vi "RegisterSettings.vi"(8 "error in":errorcluster, 11 "MainFGV_data":T1) -> (0 "error out":errorcluster, 3 "MainFGV_data out":T1)   [LabVIEW 2017]
uses:
  MainFGV_data.ctl
  CurrentMeter/CM_data.ctl
  CurrentMeter/CM_SerialNumber.ctl
  StrainGauge/SG_data.ctl
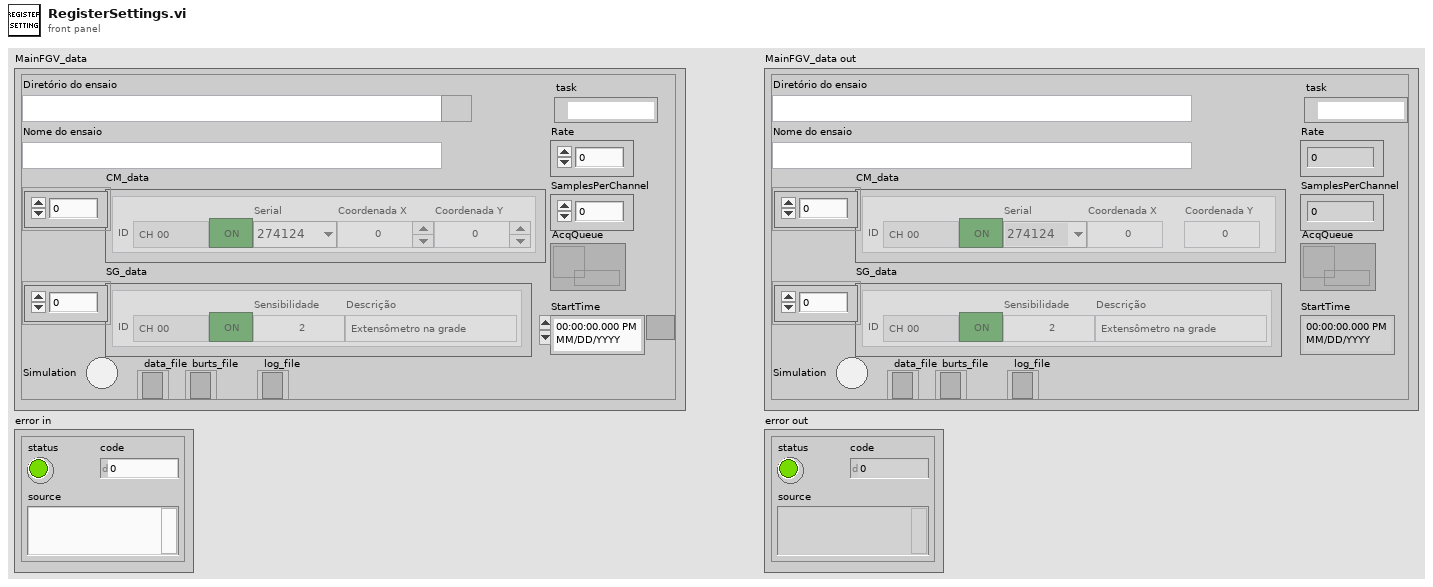
[diagram p1: front panel]
types:
  T1 = typedef "MainFGV_data.ctl" = cluster{"TestDir":path, "TestName":string, "CM_data":T2[], "SG_data":T4[], "Simulation":bool, "task":refnum<k21>, "data_file":refnum<file>, "burts_file":refnum<file>, "log_file":refnum<file>, "Rate":dbl, "SamplesPerChannel":dbl, "AcqQueue":refnum<queue>, "StartTime":timestamp}
  T2 = typedef "CM_data.ctl" = cluster{"Serial":T3, "Coordenada X":dbl, "Coordenada Y":dbl, "ID":string, "active":bool}
  T3 = typedef "CM_SerialNumber.ctl" = enum16{"274124", "274125", "274126", "274127", "274128"}
  T4 = typedef "SG_data.ctl" = cluster{"ID":string, "Sensibilidade":dbl, "Descrição":string, "active":bool}
  T5 = enum16{"open", "replace", "create", "open or create", "replace or create", "replace or create with confirmation"}
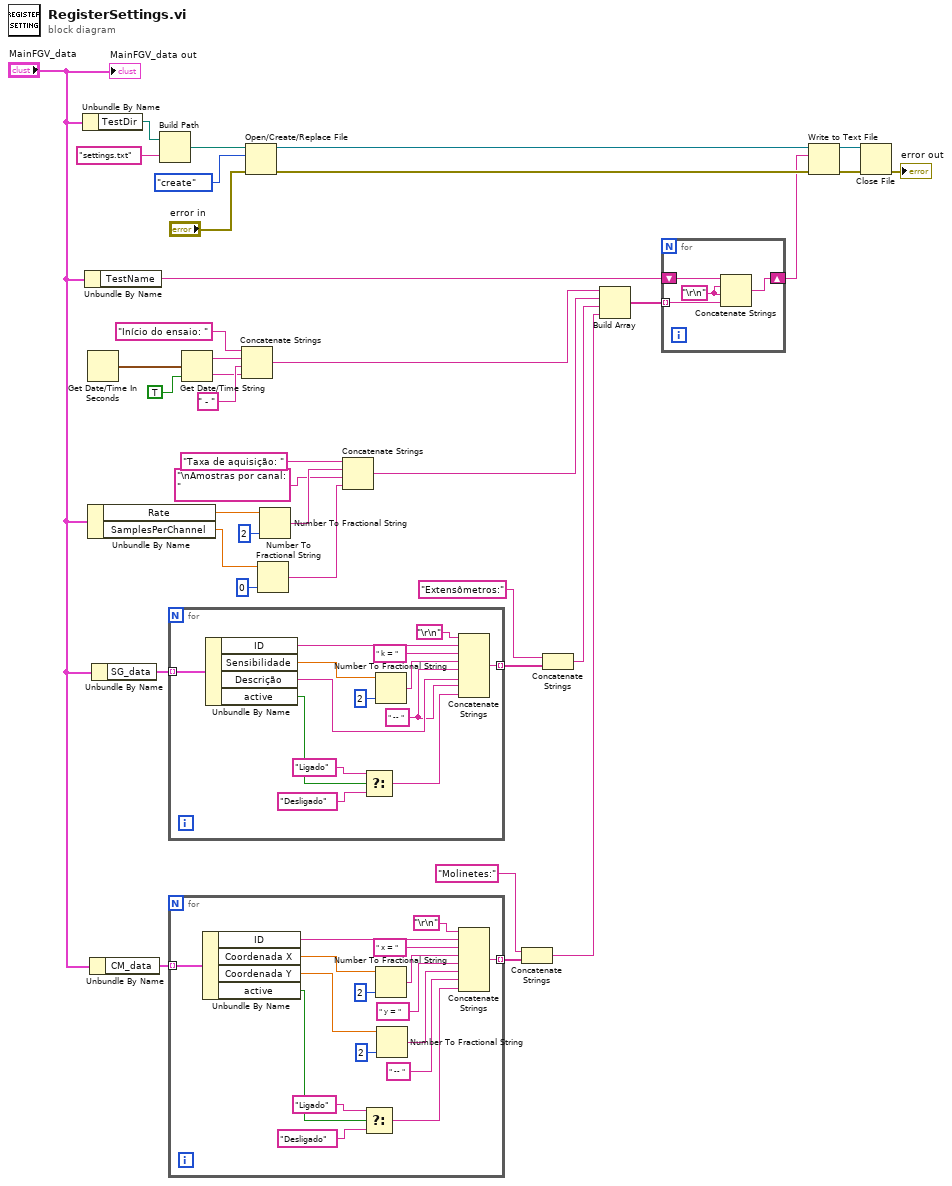
[diagram p0: block diagram]
diagram:
  n1 = Unbundle By Name("MainFGV_data") -> ("TestDir"=w38:path)
  n2 = Unbundle By Name("MainFGV_data") -> ("TestName"=w2:string)
  n3 = Get Date/Time In Seconds() -> (seconds since 1Jan1904=w1:timestamp)
  n4 = Unbundle By Name("MainFGV_data") -> ("Rate"=w28:dbl, "SamplesPerChannel"=w24:dbl)
  n5 = Unbundle By Name("MainFGV_data") -> ("CM_data"=w18:T2[])
  n6 = Unbundle By Name("MainFGV_data") -> ("SG_data"=w21:T4[])
  n7 = Build Path(base path=w38, name or relative path="settings.txt") -> (appended path=w36:path)
  n8 = for {
    tunnel: w21 -> [w52] mode=indexing
    tunnel: [w40] -> w20 mode=indexing
    w45 = " -- " ("string")
    n9 = Unbundle By Name(w52) -> ("ID"=w51:string, "Sensibilidade"=w48:dbl, "Descrição"=w46:string, "active"=w44:bool)
    n10 = Select(t="Ligado" ("string"), s=w44, f="Desligado" ("string")) -> (s? t:f=w41:string)
    n11 = Number To Fractional String(number=w48, precision (6)=i16 2) -> (F-format string=w47:string)  [unwired: 2 in]
    n12 = Concatenate Strings("\r\n", w51, " k = " ("string"), w47, w45, w46, w45, w41) -> (w40:string)
  }
  n13 = for {
    tunnel: w18 -> [w69] mode=indexing
    tunnel: [w58] -> w19 mode=indexing
    n14 = Unbundle By Name(w69) -> ("ID"=w68:string, "Coordenada X"=w65:dbl, "Coordenada Y"=w56:dbl, "active"=w62:bool)
    n15 = Select(t="Ligado" ("string"), s=w62, f="Desligado" ("string")) -> (s? t:f=w59:string)
    n16 = Number To Fractional String(number=w65, precision (6)=i16 2) -> (F-format string=w64:string)  [unwired: 2 in]
    n17 = Number To Fractional String(number=w56, precision (6)=i16 2) -> (F-format string=w55:string)  [unwired: 2 in]
    n18 = Concatenate Strings("\r\n", w68, " x = " ("string"), w64, " y = " ("string"), w55, " -- " ("string"), w59) -> (w58:string)
  }
  n19 = Get Date/Time String(seconds (now)=w1, want seconds? (F)=TRUE) -> (date string=w31:string, time string=w30:string)  [unwired: 1 in]
  n20 = Concatenate Strings("Início do ensaio: " ("string"), w31, " - " ("string"), w30) -> (w14:string)
  n21 = Open/Create/Replace File(file path (use dialog)=w36, error in="error in", operation (0:open)=T5."create") -> (refnum out=w6:refnum<file>, error out=w8:errorcluster)  [unwired: 3 in, 1 out]
  n22 = Number To Fractional String(number=w24, precision (6)=i16 0) -> (F-format string=w22:string)  [unwired: 2 in]
  n23 = Number To Fractional String(number=w28, precision (6)=i16 2) -> (F-format string=w26:string)  [unwired: 2 in]
  n24 = Concatenate Strings("Taxa de aquisição: " ("string"), w26, "\nAmostras por canal: " ("string"), w22) -> (w13:string)
  n25 = Concatenate Strings("Molinetes:" ("string"), w19) -> (w11:string)
  n26 = Concatenate Strings("Extensômetros:" ("string"), w20) -> (w12:string)
  n27 = Build Array(w14, w13, w12, w11) -> (w10:string[])
  n28 = for {
    tunnel: w10 -> [w72] mode=indexing
    shift-right: [w70] -> w7
    shift-left: w2 -> [w73]
    w71 = "\r\n"
    n29 = Concatenate Strings(w73, w71, w71, w72) -> (w70:string)
  }
  n30 = Write to Text File(file (use dialog)=w6, text=w7, error in=w8) -> (refnum out=w4:refnum<file>, error out=w5:errorcluster)  [unwired: 1 in, 1 out]
  n31 = Close File(refnum=w4, error in=w5) -> (error out=→"error out":errorcluster)  [unwired: 1 out]
  "MainFGV_data out" <- "MainFGV_data"
